vi "Pressure Calibration Top App.vi"() -> ()   [LabVIEW 2019]
uses:
  Device/Devices.ctl
panel:
  out "Boolean":bool
  out "Devices":T1
  out "data 2":cluster{"compactDAQ":tag}
  in  "btn_Shutdown":bool
  in  "tabCtl_Pressure":enum32{"Blank", "Find Devices"}(tab)
  out "bool_compactDAQ":bool
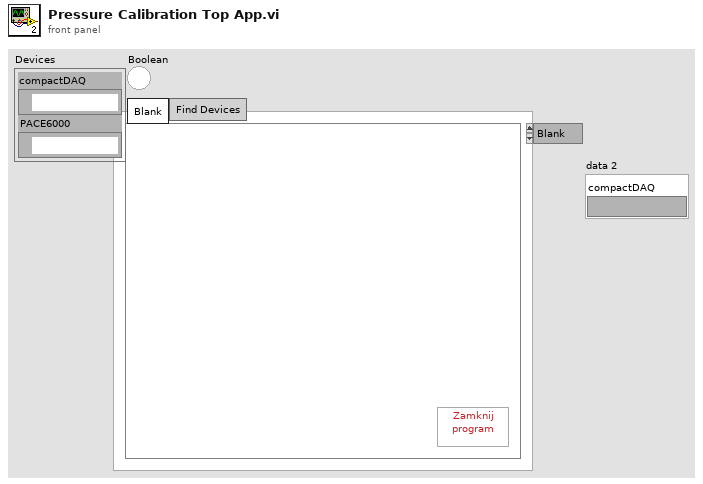
[diagram p1: front panel]
types:
  T1 = typedef "Devices.ctl" = cluster{"compactDAQ":tag, "PACE6000":refnum<visa-resource-name>}
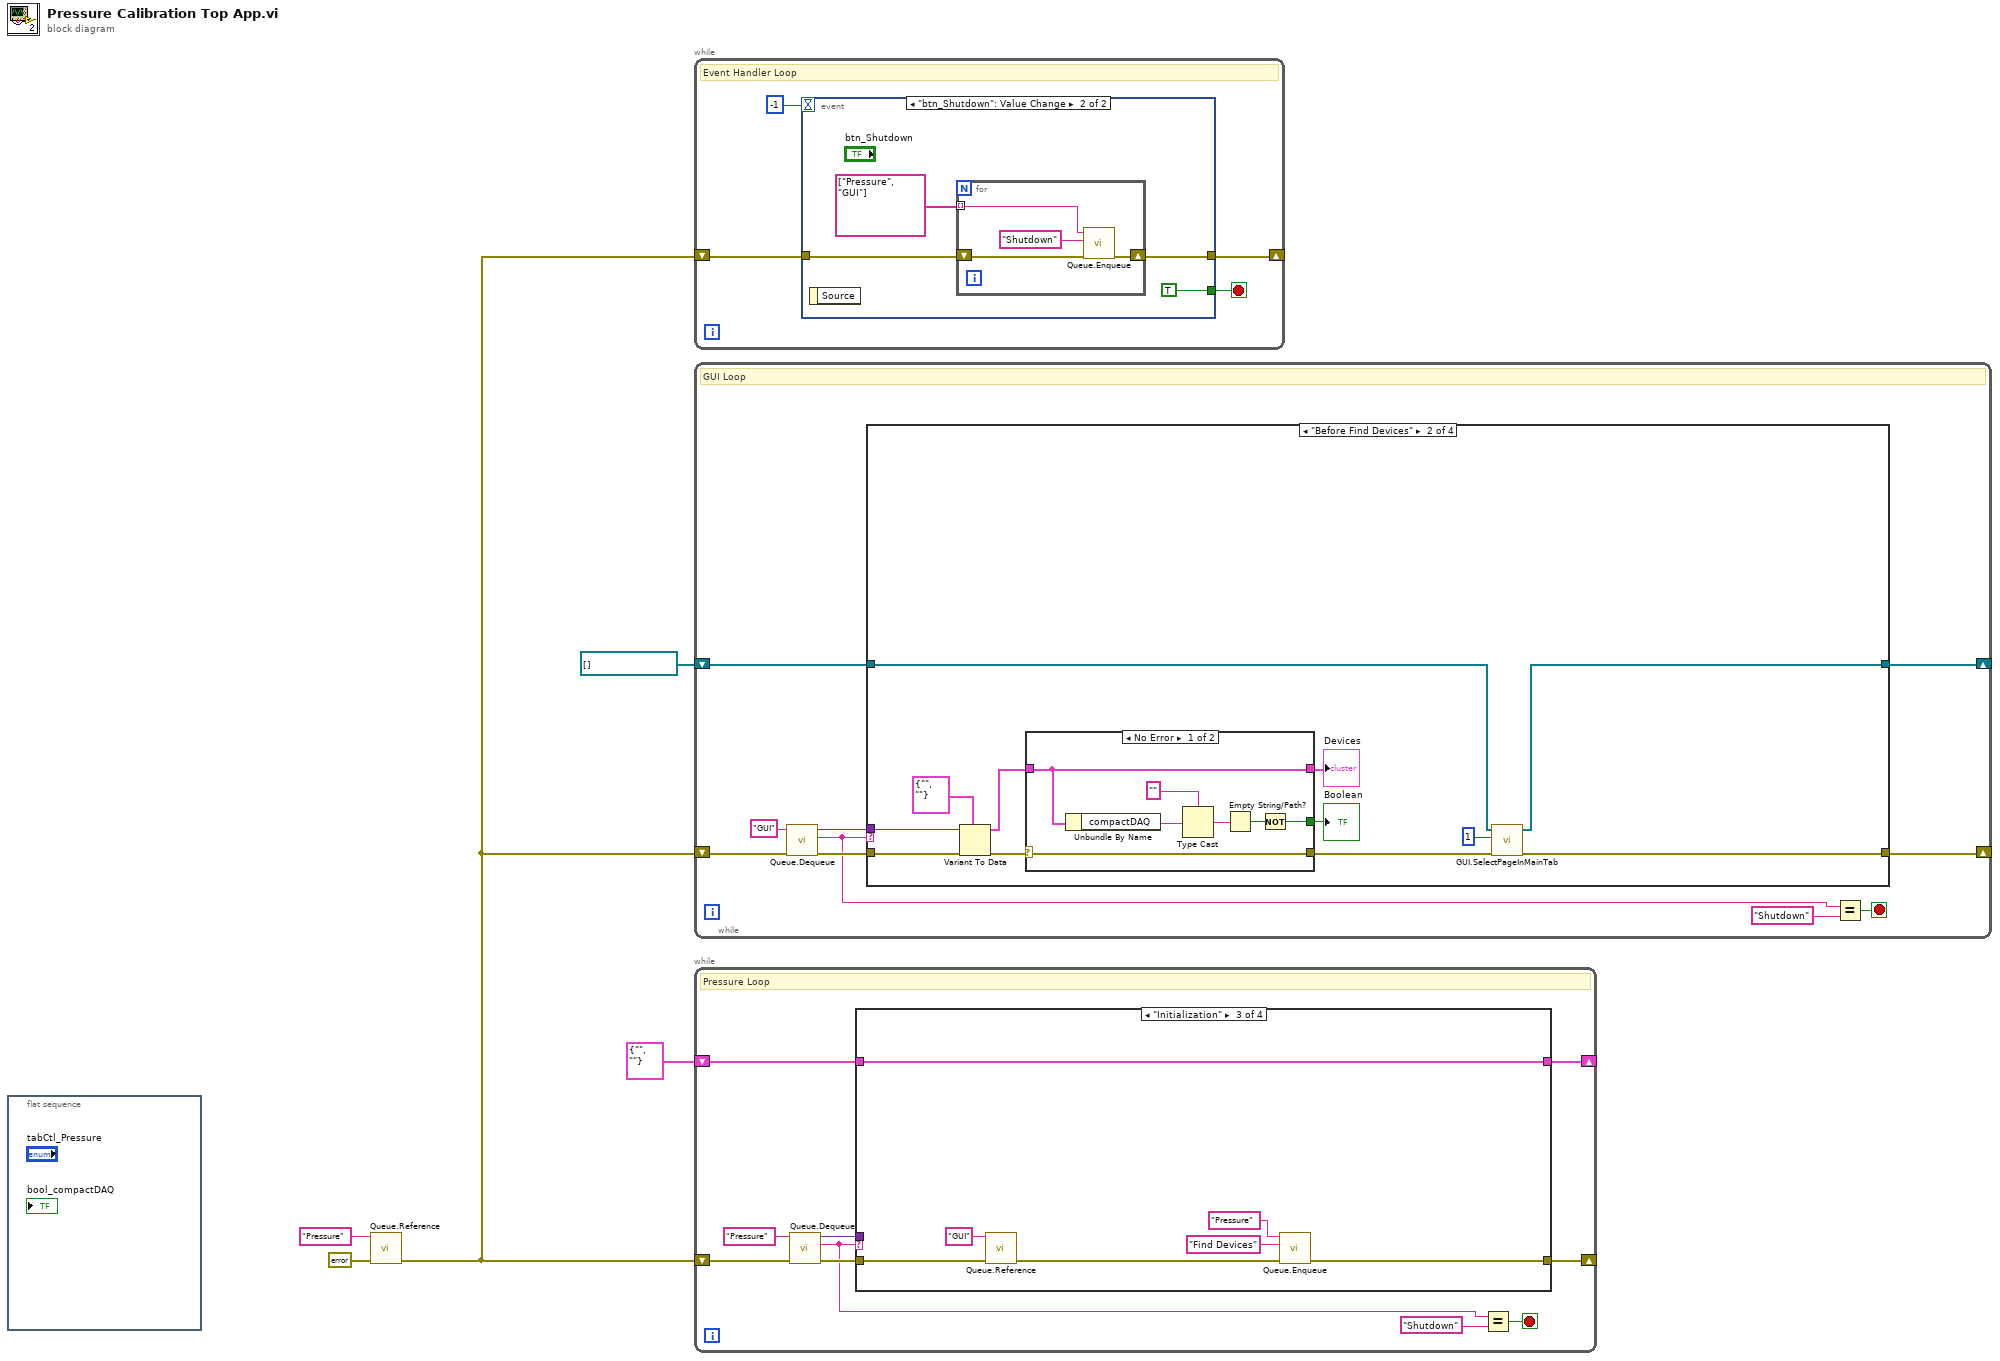
[diagram p0: block diagram]
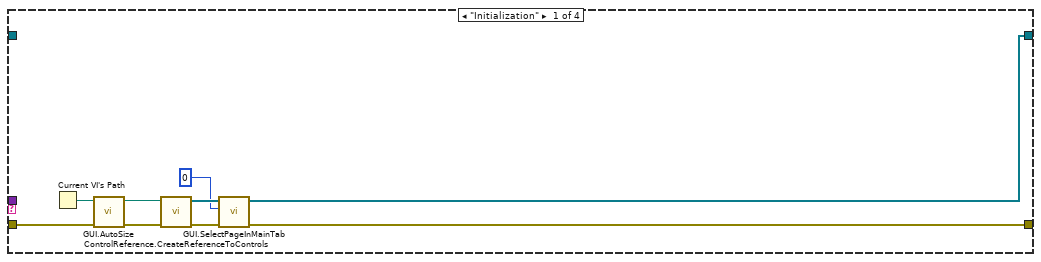
[diagram p2: hidden frame]
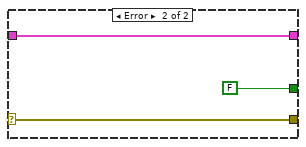
[diagram p3: hidden frame]
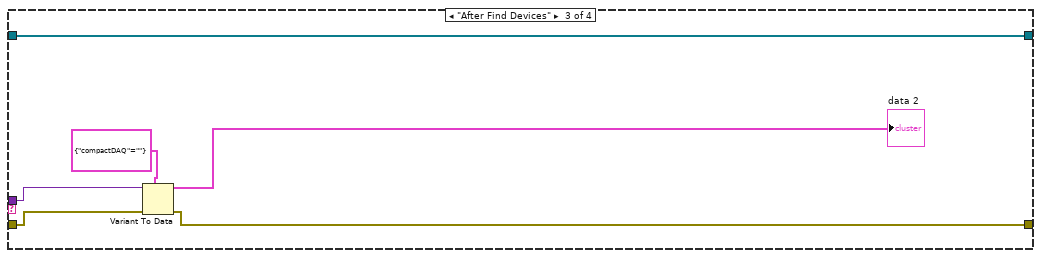
[diagram p4: hidden frame]
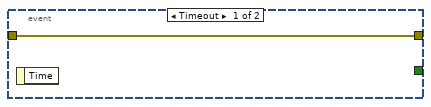
[diagram p6: hidden frame]
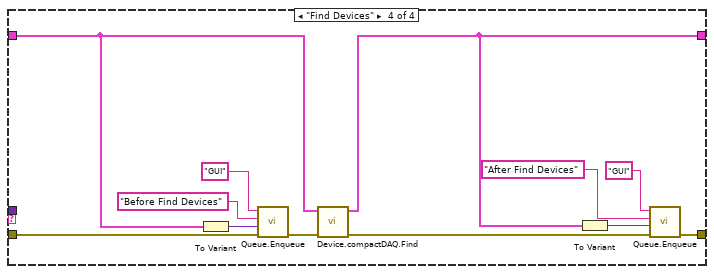
[diagram p9: hidden frame]
diagram:
  n1 = flat-sequence {
    frame #0 {
    }
  }
  n2 = call "Queue.Reference.vi"("error in (no error)"=errorcluster {"status"=FALSE, "code"=0, "source"=""} ("error constant"), "queueName"="Pressure" ("name (unnamed)")) -> ("error out"=w3:errorcluster)  [unwired: 8 in, 1 out]
  n3 = while {
    shift-right: [w7] -> _
    shift-left: w3 -> [w8]
    stop <- w6 stop-if-true
    # "Event Handler Loop"
    n4 = event shown="[1] \"btn_Shutdown\": Value Change" {
      selector: _ -> [_ _]
      dyn-events: _ -> [_ _]
      timeout: -1 -> [_ _]
      tunnel: w8 -> [w10 w13]
      tunnel: [w10 w12] -> w7
      tunnel: [_ TRUE] -> w6
      event Timeout {
        n5 = event-data() -> ()  [unwired: 1 in, 1 out]
      }
      event "btn_Shutdown": Value Change {
        n6 = event-data() -> ()  [unwired: 1 in, 1 out]
        n7 = for {
          shift-right: [w17] -> w12
          shift-left: w13 -> [w18]
          tunnel: string[] ["Pressure", "GUI"] -> [w15] mode=indexing
          n8 = call "Queue.Enqueue.vi"("error in (no error)"=w18, "message"="Shutdown", "queueName"=w15) -> ("error out"=w17:errorcluster)  [unwired: 8 in]
        }
      }
    }
  }
  n9 = while {
    shift-right: [w25] -> _
    shift-left: w3 -> [w28]
    shift-right: [w20] -> _
    shift-left: refnum<vi>[] [] ("referenceToControls") -> [w19]
    stop <- w24 stop-if-true
    # "GUI Loop"
    n10 = call "Queue.Dequeue.vi"("error in (no error)"=w28, "queueName"="GUI") -> ("error out"=w27:errorcluster, "message"=w22:string, "data"=w21:variant)  [unwired: 7 in]
    n11 = case shown="\"Before Find Devices\"" w22 {
      tunnel: w27 -> [w36 w49 w63 w67]
      tunnel: [w31 w45 w62 w67] -> w25
      tunnel: w21 -> [_ w48 w64 _]
      tunnel: [w33 w46 w60 w66] -> w20
      tunnel: w19 -> [_ w47 w60 w66]
      frame "Initialization" {
        n12 = Current VI's Path() -> (path=w37:path)
        n13 = call "GUI.AutoSize.vi"("error in (no error)"=w36, "pathToMainVI in"=w37) -> ("error out"=w35:errorcluster, "pathToMainVI out"=w34:path)  [unwired: 8 in]
        n14 = call "ControlReference.CreateReferenceToControls.vi"("error in (no error)"=w35, "pathToMainVI"=w34) -> ("error out"=w32:errorcluster, "referenceToControls"=w30:refnum<vi>[])  [unwired: 8 in]
        n15 = call "GUI.SelectPageInMainTab.vi"("error in (no error)"=w32, "pageNumber"=0, "referenceToControls in"=w30) -> ("error out"=w31:errorcluster, "referenceToControls out"=w33:refnum<vi>[])  [unwired: 7 in]
      }
      frame "Before Find Devices" {
        n16 = Variant To Data(error in=w49, type=T1 {"compactDAQ"="", "PACE6000"=""}, Variant=w48) -> (data=w42:T1, error out=w41:errorcluster)
        n17 = case shown="No Error" w41 {
          selector: w41 -> [w56 w59]
          tunnel: w42 -> [w50 w57]
          tunnel: [w56 w59] -> w40
          tunnel: [w51 FALSE] -> w38
          tunnel: [w50 w57] -> w39
          frame No Error {
            n18 = Unbundle By Name(w50) -> ("compactDAQ"=w55:tag)
            n19 = Type Cast(type="", x=w55) -> (*(type *) &x=w53:string)
            n20 = Empty String/Path?(string/path=w53) -> (empty?=w52:bool)
            n21 = Not(x=w52) -> (.not. x?=w51:bool)
          }
          frame Error {
          }
        }
        "Devices" <- w39
        "Boolean" <- w38
        n22 = call "GUI.SelectPageInMainTab.vi"("error in (no error)"=w40, "pageNumber"=1, "referenceToControls in"=w47) -> ("error out"=w45:errorcluster, "referenceToControls out"=w46:refnum<vi>[])  [unwired: 7 in]
      }
      frame "After Find Devices" {
        n23 = Variant To Data(error in=w63, type=cluster{"compactDAQ":tag} {"compactDAQ"=""}, Variant=w64) -> (data=→"data 2":cluster{"compactDAQ":tag}, error out=w62:errorcluster)
      }
      frame "Idle", Default {
      }
    }
    n24 = Equal?(x=w22, y="Shutdown") -> (x = y?=w24:bool)
  }
  n25 = while {
    shift-right: [w77] -> _
    shift-left: w3 -> [w73]
    shift-right: [w68] -> _
    shift-left: T1 {"compactDAQ"="", "PACE6000"=""} -> [w69]
    stop <- w76 stop-if-true
    # "Pressure Loop"
    n26 = call "Queue.Dequeue.vi"("error in (no error)"=w73, "queueName"="Pressure") -> ("error out"=w74:errorcluster, "message"=w72:string, "data"=w70:variant)  [unwired: 7 in]
    n27 = case shown="\"Initialization\"" w72 {
      tunnel: [w79 w81 w88 w96] -> w77
      tunnel: w74 -> [w79 w81 w84 w100]
      tunnel: w70 -> [_ _ _ _]
      tunnel: w69 -> [w78 w80 w82 w90]
      tunnel: [w78 w80 w82 w89] -> w68
      frame "Idle", Default {
      }
      frame "Shutdown" {
      }
      frame "Initialization" {
        n28 = call "Queue.Reference.vi"("error in (no error)"=w84, "queueName"="GUI" ("name (unnamed)")) -> ("error out"=w83:errorcluster)  [unwired: 8 in, 1 out]
        n29 = call "Queue.Enqueue.vi"("error in (no error)"=w83, "message"="Find Devices", "queueName"="Pressure") -> ("error out"=w88:errorcluster)  [unwired: 8 in]
      }
      frame "Find Devices" {
        n30 = To Variant(anything=w90) -> (Variant=w92:variant)
        n31 = call "Queue.Enqueue.vi"("error in (no error)"=w100, "data"=w92, "message"="Before Find Devices", "queueName"="GUI") -> ("error out"=w99:errorcluster)  [unwired: 7 in]
        n32 = call "Device.compactDAQ.Find.vi"("error in (no error)"=w99, "Devices in"=w90) -> ("error out"=w97:errorcluster, "Devices out"=w89:T1)  [unwired: 8 in]
        n33 = To Variant(anything=w89) -> (Variant=w91:variant)
        n34 = call "Queue.Enqueue.vi"("error in (no error)"=w97, "data"=w91, "message"="After Find Devices", "queueName"="GUI") -> ("error out"=w96:errorcluster)  [unwired: 7 in]
      }
    }
    n35 = Equal?(x=w72, y="Shutdown") -> (x = y?=w76:bool)
  }
